vi "_Read Config File.vi"(8 "advisory dialog? (display:T)":bool=TRUE, 10 "File Type (config)":T11, 11 "start path  (Not A Path)":path=path "") -> (0 "error":bool, 1 "Cal/Res":dbl[][](array[numeric]), 2 "Configuration":T9, 3 "new file path":path, 4 "GUI Method":T6={"Lenses"=[], "Mass Ranges"=[], "Acquire"=FALSE, "MCA"=FALSE, "Q1DC EN"=FALSE, "Q1 POL"=FALSE, "Q3 POL"=FALSE, "Q1 RF  EN"=FALSE, "Averaging"=FALSE, "Log Scale"=FALSE, "CPS"=FALSE, "Unit"=FALSE, "Data Path"=path "", "Run Mode"=enum."MRM (Q1/Q2)", "Fixed Mass (amu)"=1.0, "Q3DC EN"=FALSE, "Q3 RF  EN"=FALSE, "Negative"=FALSE} {"Mass Ranges"."Res" items=["High/High", "Medium/Medium", "Low/Low", "High/Medium", "High/Low", "Medium/High", "Medium/Low", "Low/High", "Low/Medium"]}, 5 "AcqMethod":T1[](array[typedef]) {"ScanType" format="%#.6g"; "Mass Range"."Res" items=["High/High", "Medium/Medium", "Low/Low", "High/Medium", "High/Low", "Medium/High", "Medium/Low", "Low/High", "Low/Medium"]}, 6 "Sample List":string[][](table))   [LabVIEW 2012]
uses:
  Type/_File Type.ctl
  Type/_RT Instrument 2.ctl
  Type/_RT Configuration 2.ctl
  Type/_GUI Method.ctl
  Type/_Lens Property.ctl
  Type/_Mass Range Property.ctl
  Type/_Mass Range Parameters.ctl
  Type/_RT Res Type.ctl
  Type/_Run Mode.ctl
  Type/_XML Expt.ctl
  Type/_XML Lens.ctl
  Configuration/_Global Configuration.vi
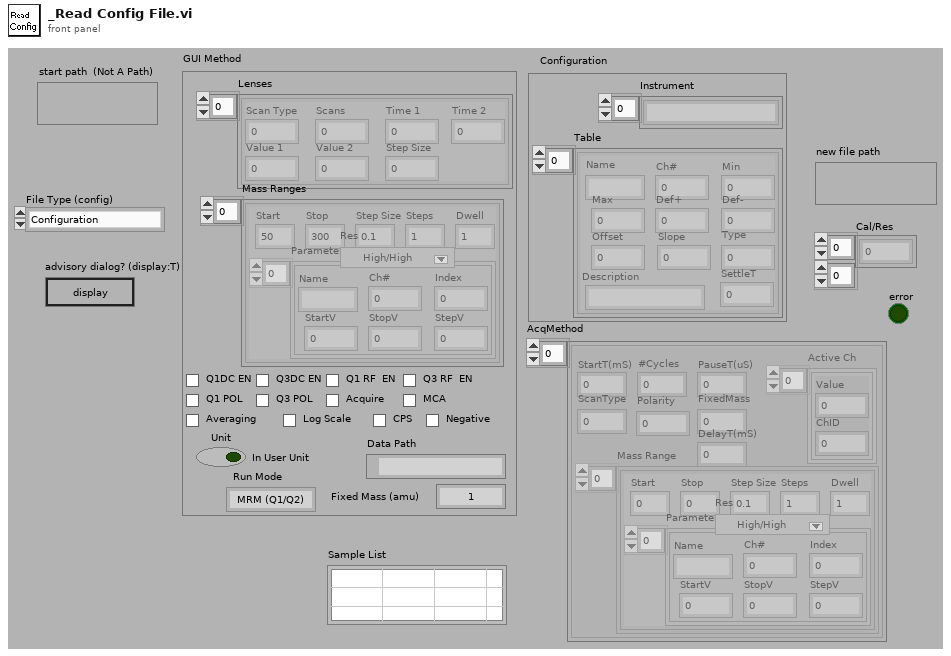
[diagram p1: front panel]
types:
  T1 = typedef "_XML Expt.ctl" = cluster{"StartT(mS)":i32, "#Cycles":i32, "PauseT(uS)":i32, "ScanType":i32, "Polarity":u8, "FixedMass":dbl, "DelayT(mS)":i32, "Active Ch":T2[], "Mass Range":T3[]}
  T2 = typedef "_XML Lens.ctl" = cluster{"Value":dbl, "ChID":u8}
  T3 = typedef "_Mass Range Property.ctl" = cluster{"Start":dbl, "Stop":dbl, "Step Size":dbl, "Steps":i32, "Dwell":dbl, "Parameters":T4[], "Res":T5}
  T4 = typedef "_Mass Range Parameters.ctl" = cluster{"Name":string, "Ch#":u8, "StartV":dbl, "StopV":dbl, "StepV":dbl, "Index":u8}
  T5 = typedef "_RT Res Type.ctl" = u16
  T6 = typedef "_GUI Method.ctl" = cluster{"Lenses":T7[], "Mass Ranges":T3[], "Acquire":bool, "MCA":bool, "Q1DC EN":bool, "Q1 POL":bool, "Q3 POL":bool, "Q1 RF  EN":bool, "Averaging":bool, "Log Scale":bool, "CPS":bool, "Unit":bool, "Data Path":path, "Run Mode":T8, "Fixed Mass (amu)":dbl, "Q3DC EN":bool, "Q3 RF  EN":bool, "Negative":bool}
  T7 = typedef "_Lens Property.ctl" = cluster{"Scan Type":u8, "Scans":i32, "Time 1":dbl, "Time 2":dbl, "Value 1":dbl, "Value 2":dbl, "Step Size":dbl}
  T8 = typedef "_Run Mode.ctl" = enum16{"MRM (Q1/Q2)", "Q1 Scan", "Q1 SRM", "Q2 Scan", "Q2 SRM", "Product Scan", "Precursor Scan", "Neutral Loss", "Neutral Gain"}
  T9 = typedef "_RT Instrument 2.ctl" = cluster{"Table":T10[], "Instrument":string[]}
  T10 = typedef "_RT Configuration 2.ctl" = cluster{"Name":string, "Ch#":u8, "Min":dbl, "Max":dbl, "Def+":dbl, "Def-":dbl, "Offset":dbl, "Slope":dbl, "Type":u8, "Description":string, "SettleT":dbl}
  T11 = typedef "_File Type.ctl" = enum16{"Configuration", "Old Configuration", "Calibration", "Resolution", "Diagnostic Method", "Old Method", "Acq Method", "Samp List"}
  T12 = cluster{"Table":cluster{"Name":string, "Ch#":u8, "Min":dbl, "Max":dbl, "Def":dbl, "Offset":dbl, "Slope":dbl, "Type":u8, "Description":string, "SettleT(nS)":u16, "Link":string}[], "Instrument":string[]}
  T13 = cluster{"Name":string, "Ch#":u8, "Min":dbl, "Max":dbl, "Def":dbl, "Offset":dbl, "Slope":dbl, "Type":u8, "Description":string, "SettleT(nS)":u16, "Link":string}[]
  T14 = cluster{"Lenses":cluster{"Scan Type":u8, "Scans":i32, "Time 1":dbl, "Time 2":dbl, "Value 1":dbl, "Value 2":dbl, "Step Size":dbl}[], "Mass Ranges":cluster{"Start":dbl, "Stop":dbl, "Step Size":dbl, "Dwell":dbl}[], "Acquire":bool, "MCA":bool, "DC EN":bool, "DC POL":bool, "MRF EN":bool, "PS EN":bool, "Averaging":bool, "Log Scale":bool, "CPS":bool, "Unit":bool, "Data Path":path, "Run Mode":T8, "Fixed Mass (amu)":dbl, "Q3DC EN":bool}
  T15 = cluster{"Start":dbl, "Stop":dbl, "Step Size":dbl, "Dwell":dbl}[]
  T16 = cluster{"Scan Type":u8, "Scans":i32, "Time 1":dbl, "Time 2":dbl, "Value 1":dbl, "Value 2":dbl, "Step Size":dbl}[]
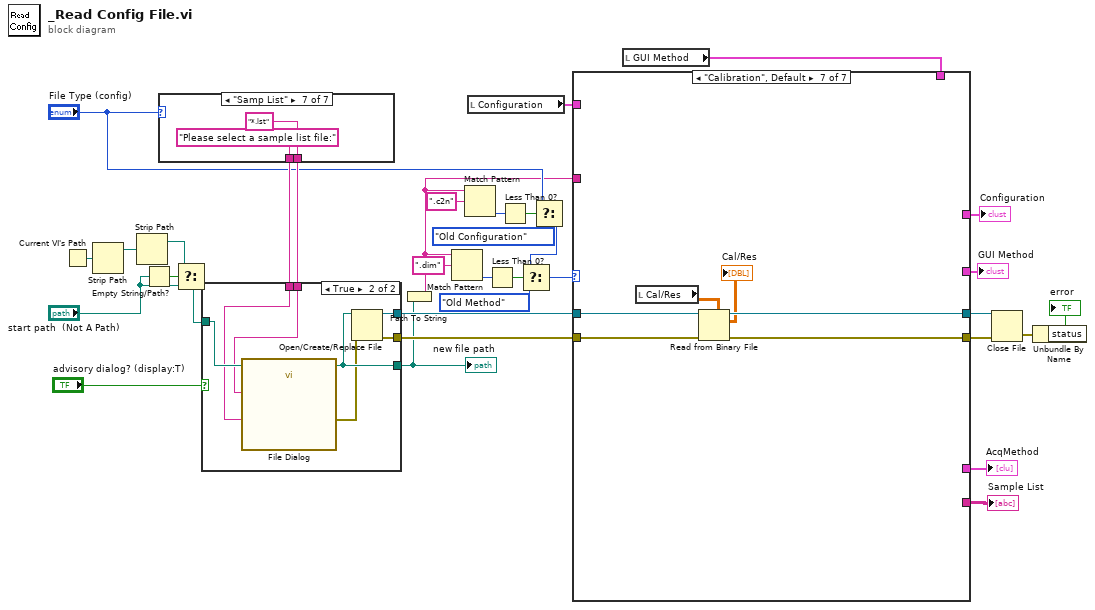
[diagram p0: block diagram]
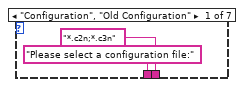
[diagram p2: hidden frame]
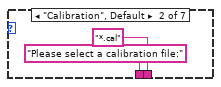
[diagram p3: hidden frame]
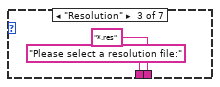
[diagram p4: hidden frame]
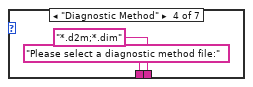
[diagram p5: hidden frame]
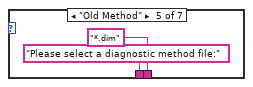
[diagram p6: hidden frame]
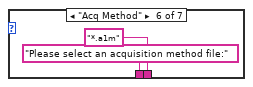
[diagram p7: hidden frame]
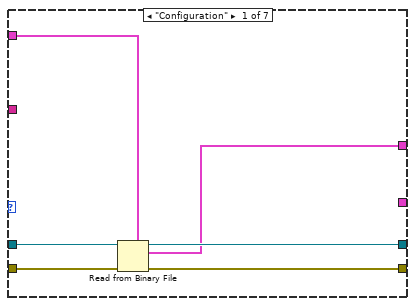
[diagram p8: hidden frame]
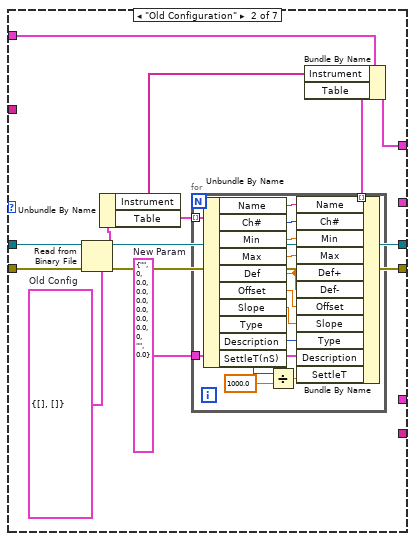
[diagram p9: hidden frame]
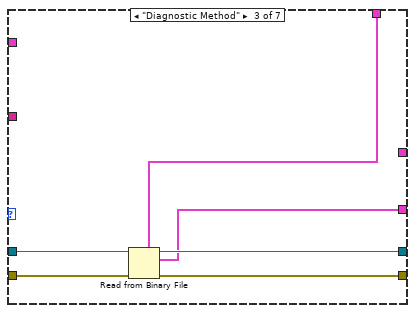
[diagram p10: hidden frame]
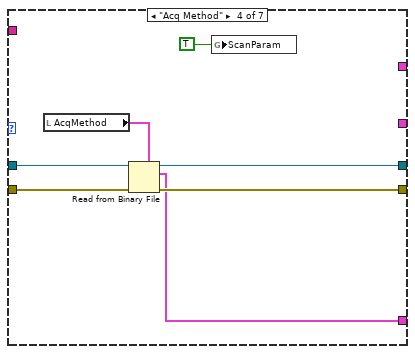
[diagram p11: hidden frame]
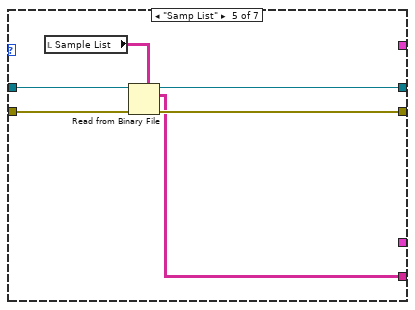
[diagram p12: hidden frame]
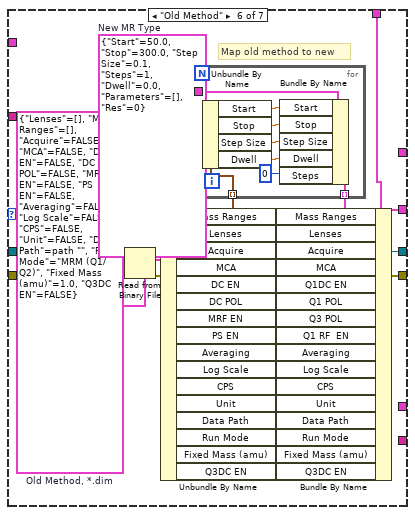
[diagram p13: hidden frame]
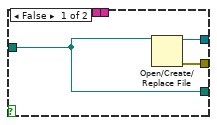
[diagram p14: hidden frame]
diagram:
  n1 = Current VI's Path() -> (path=w29:path)
  n2 = Strip Path(path=w29) -> (stripped path=w28:path)  [unwired: 1 out]
  n3 = Strip Path(path=w28) -> (stripped path=w27:path)  [unwired: 1 out]
  n4 = Empty String/Path?(string/path="start path  (Not A Path)") -> (empty?=w32:bool)
  n5 = case shown="\"Samp List\"" "File Type (config)" {
    tunnel: ["*.c2n;*.c3n" ("pattern (*.cfg)") "*.cal" ("pattern (*.cfg)") "*.res" ("pattern (*.cfg)") "*.d2m;*.dim" ("pattern (*.cfg)") "*.dim" ("pattern (*.cfg)") "*.a1m" ("pattern (*.cfg)") "*.lst" ("pattern (*.cfg)")] -> w23
    tunnel: ["Please select a configuration file:" ("prompt") "Please select a calibration file:" ("prompt") "Please select a resolution file:" ("prompt") "Please select a diagnostic method file:" ("prompt") "Please select a diagnostic method file:" ("prompt") "Please select an acquisition method file:" ("prompt") "Please select a sample list file:" ("prompt")] -> w22
    frame "Configuration", "Old Configuration" {
    }
    frame "Calibration", Default {
    }
    frame "Resolution" {
    }
    frame "Diagnostic Method" {
    }
    frame "Old Method" {
    }
    frame "Acq Method" {
    }
    frame "Samp List" {
    }
  }
  n6 = Select(t=w27, s=w32, f="start path  (Not A Path)") -> (s? t:f=w30:path)
  n7 = case shown="True" "advisory dialog? (display:T)" {
    tunnel: w22 -> [_ w57]
    tunnel: w23 -> [_ w52]
    tunnel: [w49 w54] -> w19
    tunnel: [w51 w56] -> w34
    tunnel: [w50 w55] -> w33
    tunnel: w30 -> [w49 w58]
    frame False {
      n8 = Open/Create/Replace File(file path (use dialog)=w49) -> (refnum out=w51:refnum<file>, error out=w50:errorcluster)  [unwired: 5 in, 1 out]
    }
    frame True {
      n9 = call "File Dialog"("start path"=w58, "prompt"=w57, "pattern (all files)"=w52) -> ("selected path"=w54:path, "error out"=w53:errorcluster)  [unwired: 9 in, 2 out]
      n10 = Open/Create/Replace File(file path (use dialog)=w54, error in=w53) -> (refnum out=w56:refnum<file>, error out=w55:errorcluster)  [unwired: 4 in, 1 out]
    }
  }
  "new file path" <- w19
  n11 = Path To String(path=w19) -> (string=w5:string)
  n12 = Match Pattern(string=w5, regular expression=".dim") -> (offset past match=w17:i32)  [unwired: 4 out]
  n13 = Match Pattern(string=w5, regular expression=".c2n") -> (offset past match=w13:i32)  [unwired: 4 out]
  n14 = local read "Configuration"() -> (w7:T9)
  n15 = Less Than 0?(x=w17) -> (x < 0?=w16:bool)
  n16 = Less Than 0?(x=w13) -> (x < 0?=w14:bool)
  n17 = Select(t="File Type (config)", s=w14, f=_File_Type."Old Configuration") -> (s? t:f=w9:T11)
  n18 = Select(t=w9, s=w16, f=_File_Type."Old Method") -> (s? t:f=w8:T11)
  n19 = local read "GUI Method"() -> (w20:T6)
  n20 = case shown="\"Calibration\", Default" w8 {
    tunnel: w34 -> [w64 w76 w97 w104 w110 w136 w150]
    tunnel: w33 -> [w63 w75 w96 w103 w109 w135 w149]
    tunnel: [w62 w74 w95 w102 w108 w134 w148] -> w25
    tunnel: [w61 w73 w94 w101 w107 w133 w147] -> w24
    tunnel: [_ _ w93 _ _ w111 _] -> w21
    tunnel: w20 -> [_ _ w92 _ _ w130 _]
    tunnel: w7 -> [w60 w71 _ _ _ _ _]
    tunnel: [w59 w70 _ _ _ _ _] -> w6
    tunnel: w5 -> [_ _ _ _ _ _ _]
    tunnel: [_ _ _ w99 _ _ _] -> w4
    tunnel: [_ _ _ _ w105 _ _] -> w3
    frame "Configuration" {
      n21 = Read from Binary File(5:w60, 8:w63, 11:w64) -> (0:w61:errorcluster, 2:w59:T9, 3:w62:refnum<file>)  [unwired: 4 out]
    }
    frame "Old Configuration" {
      w66 = T12 {"Table"=[], "Instrument"=[]}  # Old Config
      w68 = T10 {"Name"="", "Ch#"=0, "Min"=0.0, "Max"=0.0, "Def+"=0.0, "Def-"=0.0, "Offset"=0.0, "Slope"=0.0, "Type"=0, "Description"="", "SettleT"=0.0}  # New Param
      n22 = Read from Binary File(5:w66, 8:w75, 11:w76) -> (0:w73:errorcluster, 2:w72:T12, 3:w74:refnum<file>)  [unwired: 4 out]
      n23 = Unbundle By Name(w72) -> ("Instrument"=w65:string[], "Table"=w69:T13)
      n24 = for {
        tunnel: w69 -> [w91] mode=indexing
        tunnel: w68 -> [w90]
        tunnel: [w85] -> w67 mode=indexing
        n25 = Unbundle By Name(w91) -> ("Name"=w89:string, "Ch#"=w88:u8, "Min"=w87:dbl, "Max"=w86:dbl, "Def"=w80:dbl, "Offset"=w81:dbl, "Slope"=w82:dbl, "Type"=w83:u8, "Description"=w84:string, "SettleT(nS)"=w79:u16)
        n26 = Divide(x=w79, y=1000.0) -> (x/y=w77:dbl)
        n27 = Bundle By Name(cluster=w90, "Name"=w89, "Ch#"=w88, "Min"=w87, "Max"=w86, "Def+"=w80, "Def-"=w80, "Offset"=w81, "Slope"=w82, "Type"=w83, "Description"=w84, "SettleT"=w77) -> (w85:T10)
      }
      n28 = Bundle By Name(cluster=w71, "Instrument"=w65, "Table"=w67) -> (w70:T9)
    }
    frame "Diagnostic Method" {
      n29 = Read from Binary File(5:w92, 8:w96, 11:w97) -> (0:w94:errorcluster, 2:w93:T6, 3:w95:refnum<file>)  [unwired: 4 out]
    }
    frame "Acq Method" {
      n30 = local read "AcqMethod"() -> (w100:T1[])
      n31 = Read from Binary File(5:w100, 8:w103, 11:w104) -> (0:w101:errorcluster, 2:w99:T1[], 3:w102:refnum<file>)  [unwired: 4 out]
      n32 = global write "_Global Configuration.vi" "ScanParam"(TRUE ("ScanParam")) -> ()
    }
    frame "Samp List" {
      n33 = local read "Sample List"() -> (w106:string[][])
      n34 = Read from Binary File(5:w106, 8:w109, 11:w110) -> (0:w107:errorcluster, 2:w105:string[][], 3:w108:refnum<file>)  [unwired: 4 out]
    }
    frame "Old Method" {
      w113 = T3 {"Start"=50.0, "Stop"=300.0, "Step Size"=0.1, "Steps"=1, "Dwell"=0.0, "Parameters"=[], "Res"=0}  # New MR Type
      w132 = T14 {"Lenses"=[], "Mass Ranges"=[], "Acquire"=FALSE, "MCA"=FALSE, "DC EN"=FALSE, "DC POL"=FALSE, "MRF EN"=FALSE, "PS EN"=FALSE, "Averaging"=FALSE, "Log Scale"=FALSE, "CPS"=FALSE, "Unit"=FALSE, "Data Path"=path "", "Run Mode"=enum."MRM (Q1/Q2)", "Fixed Mass (amu)"=1.0, "Q3DC EN"=FALSE}  # Old Method, *.dim
      # "Map old method to new"
      n35 = Read from Binary File(5:w132, 8:w135, 11:w136) -> (0:w133:errorcluster, 2:w131:T14, 3:w134:refnum<file>)  [unwired: 4 out]
      n36 = Unbundle By Name(w131) -> ("Mass Ranges"=w114:T15, "Lenses"=w115:T16, "Acquire"=w116:bool, "MCA"=w117:bool, "DC EN"=w118:bool, "DC POL"=w119:bool, "MRF EN"=w120:bool, "PS EN"=w121:bool, "Averaging"=w122:bool, "Log Scale"=w123:bool, "CPS"=w124:bool, "Unit"=w125:bool, "Data Path"=w126:path, "Run Mode"=w127:T8, "Fixed Mass (amu)"=w128:dbl, "Q3DC EN"=w129:bool)
      n37 = for {
        tunnel: w114 -> [w144] mode=indexing
        tunnel: w113 -> [w142]
        tunnel: [w138] -> w112 mode=indexing
        n38 = Unbundle By Name(w144) -> ("Start"=w143:dbl, "Stop"=w141:dbl, "Step Size"=w140:dbl, "Dwell"=w139:dbl)
        n39 = Bundle By Name(cluster=w142, "Start"=w143, "Stop"=w141, "Step Size"=w140, "Dwell"=w139, "Steps"=0) -> (w138:T3)
      }
      n40 = Bundle By Name(cluster=w130, "Mass Ranges"=w112, "Lenses"=w115, "Acquire"=w116, "MCA"=w117, "Q1DC EN"=w118, "Q1 POL"=w119, "Q3 POL"=w120, "Q1 RF  EN"=w121, "Averaging"=w122, "Log Scale"=w123, "CPS"=w124, "Unit"=w125, "Data Path"=w126, "Run Mode"=w127, "Fixed Mass (amu)"=w128, "Q3DC EN"=w129) -> (w111:T6)
    }
    frame "Calibration", Default {
      n41 = local read "Cal/Res"() -> (w146:dbl[][])
      n42 = Read from Binary File(5:w146, 8:w149, 11:w150) -> (0:w147:errorcluster, 2:→"Cal/Res":dbl[][], 3:w148:refnum<file>)  [unwired: 4 out]
    }
  }
  "GUI Method" <- w21
  "Configuration" <- w6
  "AcqMethod" <- w4
  "Sample List" <- w3
  n43 = Close File(refnum=w25, error in=w24) -> (error out=w2:errorcluster)  [unwired: 1 out]
  n44 = Unbundle By Name(w2) -> ("status"=→"error":bool)
